vi "QE Read N Chans.vi"(8 "Error In":errorcluster, 10 "QE Channel(s)":u8[](array[numeric]), 11 "LINX Resource":T1) -> (0 "Error Out":errorcluster, 2 "QE Counters":i32[](array[numeric]), 3 "LINX Resource":T1)   [LabVIEW 2013, in "LVH-LINX.lvlib"]
doc: "Read the counter values of the specified quadrature encoder channels."
uses:
  LVH-LINX.lvlib
  Private/Type Defs/LINX Ref.ctl
  Private/Type Defs/Platform.ctl
  Private/Type Defs/Interface.ctl
  Private/Device/Type Defs/LINX Device Config.ctl
  Private/Device/Type Defs/TCP Config.ctl
  Private/Device/Type Defs/Channels.ctl
  Private/Type Defs/Peripheral.ctl
  Private/Type Defs/Error Type.ctl
  Private/myRIO/myRIO.lvlib
  Private/Device/Device.lvlib
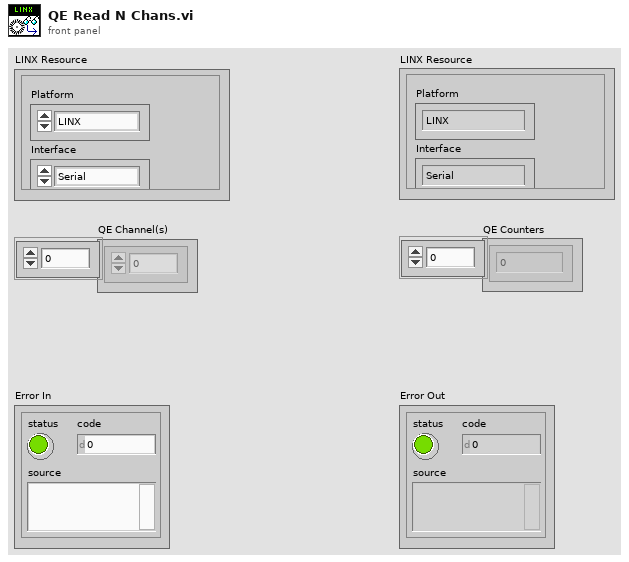
[diagram p1: front panel]
types:
  T1 = typedef "LVH-LINX.lvlib/LINX Ref.ctl" = cluster{"Platform":T2, "Interface":T3, "LINX Device Config":T4}
  T2 = typedef "LVH-LINX.lvlib/Platform.ctl" = enum16{"LINX", "myRIO"}
  T3 = typedef "LVH-LINX.lvlib/Interface.ctl" = enum16{"Serial", "TCP"}
  T4 = typedef "LVH-LINX.lvlib/Device.lvlib/LINX Device Config.ctl" = cluster{"Interface":T3, "COM Port":refnum<visa-resource-name>, "TCP Configuration":T5, "Device Family":u8, "Device ID":u8, "Device Name":string, "TCP Ref":refnum<k5>, "Channels":T6}
  T5 = typedef "LVH-LINX.lvlib/Device.lvlib/TCP Config.ctl" = cluster{"IP Address":string, "Port":u16}
  T6 = typedef "LVH-LINX.lvlib/Channels.ctl" = cluster{"DI Channels":u8[], "DO Channels":u8[], "AI":u8[], "AO":u8[], "PWM":u8[], "QE":u8[], "UART":u8[], "I2C 2":u8[], "SPI":u8[], "CAN":u8[], "AI Ref (V)":dbl, "AO Resolution (Bits)":u8, "AO Ref (V)":dbl}
  T7 = typedef "LVH-LINX.lvlib/Peripheral.ctl" = enum8{"DI", "DO", "AI", "AO", "PWM", "QE", "UART", "I2C", "SPI", "CAN"}
  T8 = typedef "LVH-LINX.lvlib/Error Type.ctl" = enum16{"Unknown", "Timeout", "Corrupt Return Packet", "Unable To Connect", "Command Not Supported", "Channel DNE", "Invalid COM Config", "Firmware Version Mismatch", "myRIO Support"}
  T9 = typedef "AI.lvlib/AI Reference.ctl" = cluster{"myRIO Reference":T10, "AI Channels List":T14, "AI Scaling Constants List":T16}
  T10 = typedef "myRIO Generic Hardware Reference.ctl" = cluster{"myRIO Model":T11, "myRIO Hardware Reference":T12}
  T11 = typedef "Hardware Version Enum.ctl" = enum16{"Unknown", "myRIO-1900", "myRIO-1950"}
  T12 = typedef "myRIO v1.0 Reference.ctl" = cluster{"Generic FPGA Reference":T13, "Allow multiple opens":bool}
  T13 = typedef "Generic FPGA Reference.ctl" = refnum<k20>
  T14 = typedef "AI Channels List.ctl" = T15[]
  T15 = typedef "AI Channels Enum.ctl" = enum16{"Not Connected", "AudioIn/Left", "AudioIn/Right", "C/AI0", "C/AI1", "A/AI0", "A/AI1", "A/AI2", "A/AI3", "B/AI0", "B/AI1", "B/AI2", "B/AI3"}
  T16 = typedef "Analog Scaling Constants List.ctl" = T17[]
  T17 = typedef "Analog Scaling Constants.ctl" = cluster{"LSB Weight (Volts)":dbl, "Offset (Volts)":dbl, "Signed?":bool}
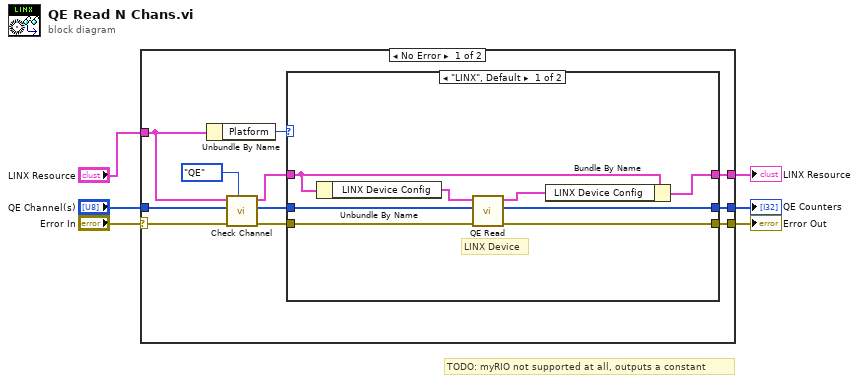
[diagram p0: block diagram]
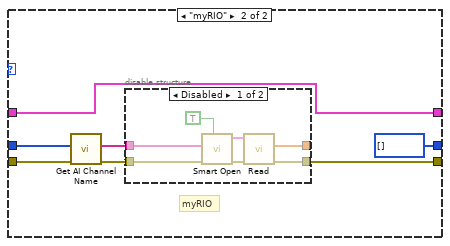
[diagram p2: hidden frame]
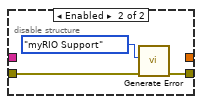
[diagram p3: hidden frame]
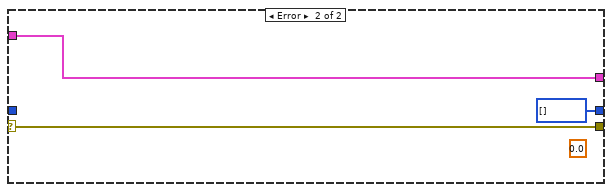
[diagram p4: hidden frame]
diagram:
  # "TODO: myRIO not supported at all, outputs a constant"
  n1 = case shown="No Error" "Error In" {
    selector: "Error In" -> [w8 w45]
    tunnel: [w16 w45] -> w6
    tunnel: [w15 w44] -> w5
    tunnel: "LINX Resource" -> [w10 w44]
    tunnel: "QE Channel(s)" -> [w9 _]
    tunnel: [w7 i32[] [] ("Counters")] -> w1
    frame No Error {
      n2 = Unbundle By Name(w10) -> ("Platform"=w17:T2)
      n3 = call "Check Channel.vi"("Peripheral"=Peripheral."QE", "Error In"=w8, "Channels"=w9, "LINX Resource"=w10) -> ("Error Out"=w14:errorcluster, "Channels"=w13:u8[], "LINX Resource"=w11:T1)  [unwired: 5 in]
      n4 = case shown="\"LINX\", Default" w17 {
        tunnel: w14 -> [w18 w28]
        tunnel: w11 -> [w25 w32]
        tunnel: [w20 w30] -> w16
        tunnel: [w24 w32] -> w15
        tunnel: w13 -> [w19 w31]
        tunnel: [w21 i32[] [] ("Counters")] -> w7
        frame "LINX", Default {
          # "LINX Device"
          n5 = Unbundle By Name(w25) -> ("LINX Device Config"=w23:T4)
          n6 = call "QE Read.vi"("Error In"=w18, "QE Channels"=w19, "LINX Device Config"=w23) -> ("Error Out"=w20:errorcluster, "Counters"=w21:i32[], "LINX Device Config"=w22:T4)  [unwired: 6 in]
          n7 = Bundle By Name(cluster=w25, "LINX Device Config"=w22) -> (w24:T1)
        }
        frame "myRIO" {
          # "myRIO"
          n8 = call "Get AI Channel Name.vi"("Error In"=w28, "AI Channel Nums"=w31) -> ("Error Out"=w27:errorcluster, "AI Channels"=w29:string[])  [unwired: 7 in]
          n9 = disable-structure shown="Disabled" {
            disable-tunnel: w27 -> [w37 w42]
            disable-tunnel: [w36 w41] -> w30
            disable-tunnel: w29 -> [w34 _]
            disable-tunnel: [w33 _] -> _
            frame Disabled {
              n10 = call <vilib>:"Smart Open.vi"("Allow multiple opens?"=TRUE, "error in (no error)"=w37, "Channel Names"=w34) -> ("error out"=w39:errorcluster, "AI Ref Out"=w38:T9)  [unwired: 7 in]
              n11 = call <vilib>:"Read.vi"("error in (no error)"=w39, "AI Ref In"=w38) -> ("error out"=w36:errorcluster, "Values"=w33:dbl[])  [unwired: 7 in, 1 out]
            }
            frame Enabled {
              n12 = call "Generate Error.vi"("Error In"=w42, "Error Type"=Error_Type."myRIO Support") -> ("Error Out"=w41:errorcluster)  [unwired: 8 in, 1 out]
            }
          }
        }
      }
    }
    frame Error {
      (unwired) 0.0 ("AI Ref")
    }
  }
  "Error Out" <- w6
  "LINX Resource" <- w5
  "QE Counters" <- w1
